vi "test2-ErrorStr conversion.vi"(8 "error in (no error)":errorcluster, 11 "TestCase in":refnum<class "testcase-CSMArgument.lvclass">) -> (0 "error out":errorcluster, 3 "TestCase out":refnum<class "testcase-CSMArgument.lvclass">)   [LabVIEW 2017, in "testcase-CSMArgument.lvclass"]
uses:
  testcase-CSMArgument.lvclass
  src/user.lib/_NEVSTOP/Communicable State Machine(CSM)/AdvanceAPI/CSM - Revert Arguments-Safe String.vi
  src/user.lib/_NEVSTOP/Communicable State Machine(CSM)/AdvanceAPI/CSM - Make String Arguments Safe.vi
  src/user.lib/_NEVSTOP/Communicable State Machine(CSM)/AdvanceAPI/CSM - Keywords.vi
  src/user.lib/_NEVSTOP/Communicable State Machine(CSM)/_Shared/Trim Single-line Text.vi
  <vilib>/addons/_JKI Toolkits/VI Tester/TestCase.llb/TestCase.lvclass
  src/user.lib/_NEVSTOP/Communicable State Machine(CSM)/Communicable State Machine.lvlib
  src/user.lib/_NEVSTOP/Communicable State Machine(CSM)/_Shared/CSM Shared.lvlib
  C:/Program Files (x86)/National Instruments/LabVIEW 2017/vi.lib/addons/_JKI Toolkits/VI Tester/TestCase.llb/TestCase.lvclass
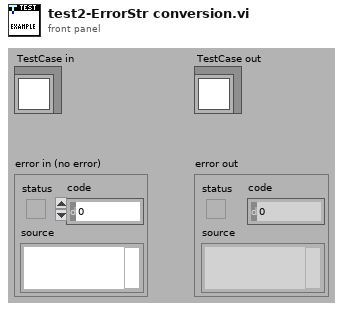
[diagram p1: front panel]
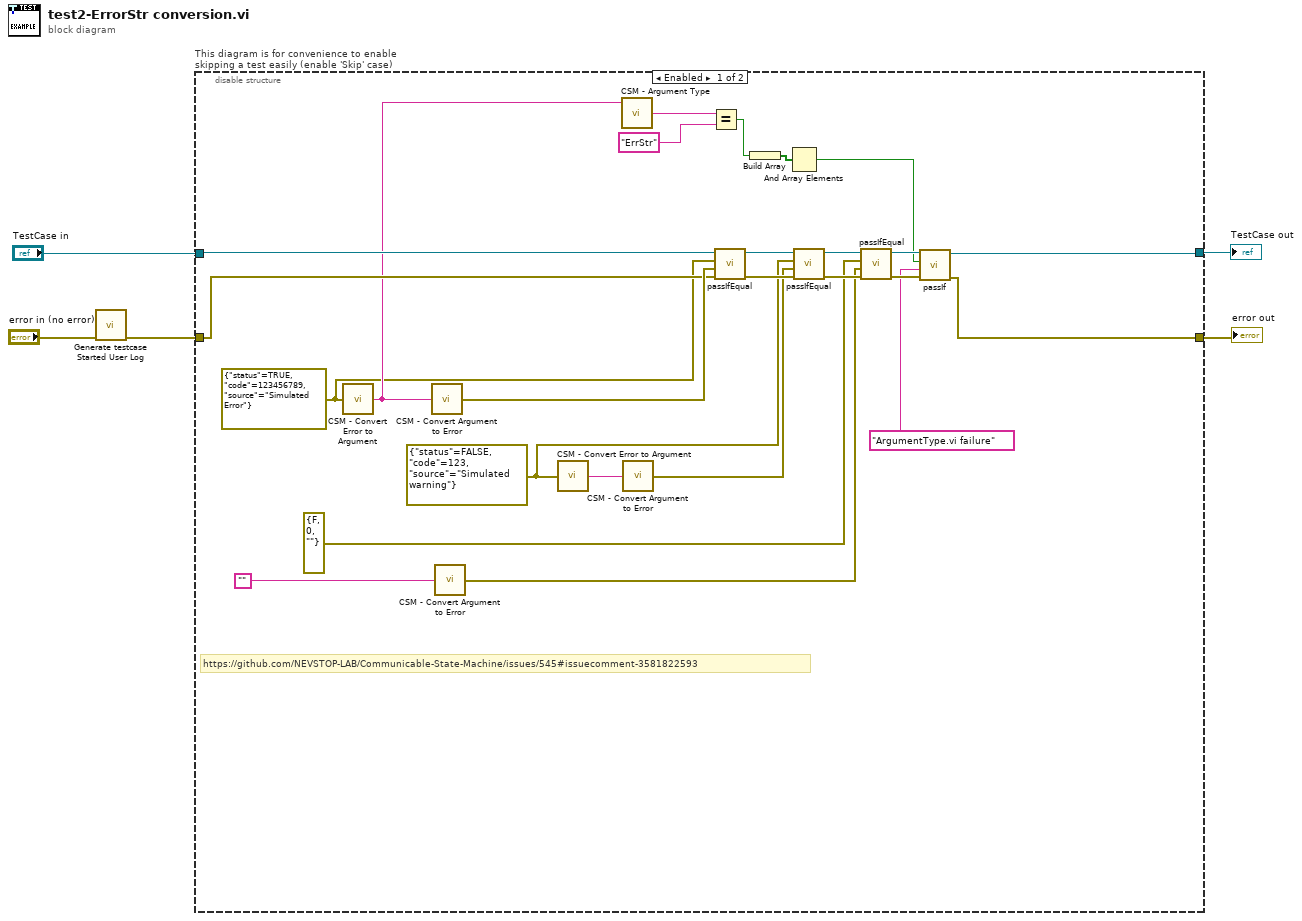
[diagram p0: block diagram]
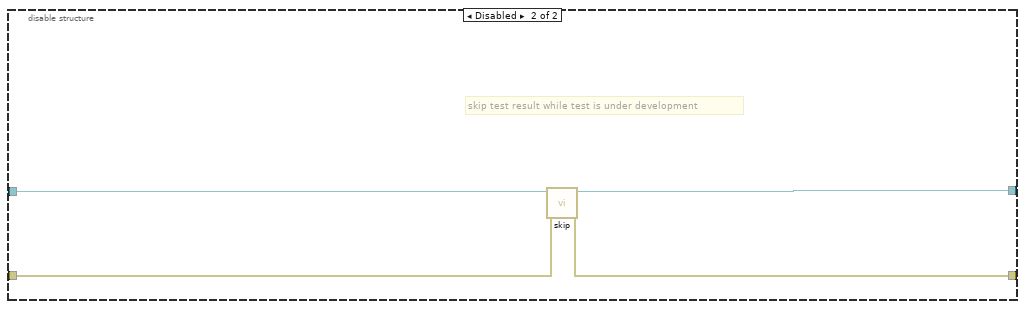
[diagram p2: hidden frame]
diagram:
  n1 = call "Generate testcase Started User Log.vi"("Error In"="error in (no error)") -> ("error out"=w1:errorcluster)  [unwired: 10 in]
  n2 = disable-structure "This diagram is for convenience to enable skipping a test easily (enable 'Skip' case)" shown="Enabled" {
    disable-tunnel: "TestCase in" -> [w30 w34]
    disable-tunnel: [w12 w32] -> w2
    disable-tunnel: [w14 w33] -> w4
    disable-tunnel: w1 -> [w24 w31]
    frame Enabled {
      w8 = errorcluster {"status"=FALSE, "code"=123, "source"="Simulated warning"} ("error constant")
      w6 = errorcluster {"status"=TRUE, "code"=123456789, "source"="Simulated Error"} ("error constant")
      # "https://github.com/NEVSTOP-LAB/Communicable-State-Machine/issues/545#issuecomment-3581822593"
      n3 = call "CSM - Convert Error to Argument.vi"("Error"=w6) -> ("Argument"=w17:string)  [unwired: 4 in]
      n4 = call "CSM - Convert Argument to Error.vi"("Argument"=w17) -> ("Error"=w25:errorcluster)  [unwired: 4 in]
      n5 = call "CSM - Convert Argument to Error.vi"("Argument"="") -> ("Error"=w21:errorcluster)  [unwired: 4 in]
      n6 = call "CSM - Convert Error to Argument.vi"("Error"=w8) -> ("Argument"=w16:string)  [unwired: 4 in]
      n7 = call "CSM - Argument Type.vi"("Arguments"=w17) -> ("Argument Type"=w18:string)  [unwired: 3 in, 1 out]
      n8 = call "CSM - Convert Argument to Error.vi"("Argument"=w16) -> ("Error"=w23:errorcluster)  [unwired: 4 in]
      n9 = Equal?(x=w18, y="ErrStr") -> (x = y?=w20:bool)
      n10 = call-dynamic "passIfEqual.vi"("error in (no error)"=w24, "y"=w25, "x"=w6, "TestCase in"=w30) -> ("error out"=w28:errorcluster, "TestCase out"=w29:refnum<class "testcase-CSMArgument.lvclass">)  [unwired: 6 in]
      n11 = Build Array(w20) -> (w19:bool[])
      n12 = And Array Elements(Boolean array=w19) -> (logical AND=w11:bool)
      n13 = call-dynamic "passIfEqual.vi"("error in (no error)"=w28, "y"=w23, "x"=w8, "TestCase in"=w29) -> ("error out"=w26:errorcluster, "TestCase out"=w27:refnum<class "testcase-CSMArgument.lvclass">)  [unwired: 6 in]
      n14 = call-dynamic "passIfEqual.vi"("error in (no error)"=w26, "y"=w21, "x"=errorcluster {"status"=FALSE, "code"=0, "source"=""} ("error constant"), "TestCase in"=w27) -> ("error out"=w15:errorcluster, "TestCase out"=w13:refnum<class "testcase-CSMArgument.lvclass">)  [unwired: 6 in]
      n15 = call-dynamic "passIf.vi"("error in (no error)"=w15, "message (\"\")"="ArgumentType.vi failure" ("message (\"\")"), "pass"=w11, "TestCase in"=w13) -> ("error out"=w14:errorcluster, "TestCase out"=w12:refnum<class "testcase-CSMArgument.lvclass">)  [unwired: 6 in]
    }
    frame Disabled {
      # "skip test result while test is under development"
      n16 = call <vilib>:"skip.vi"("error in (no error)"=w31, "TestCase in"=w34) -> ("error out"=w33:errorcluster, "TestCase out"=w32:refnum<class "testcase-CSMArgument.lvclass">)  [unwired: 8 in]
    }
  }
  "error out" <- w4
  "TestCase out" <- w2
